vi "FPGA.vi"() -> ()   [LabVIEW 2014]
uses:
  <vilib>/eio/EIONode/EIONode.xnode
  <vilib>/rvi/eio/common/nirviEmuTemplateMethod_errors.vi
panel:
  out "AI5":fxp<+/-,24,5>
  out "AI4":fxp<+/-,24,5>
  out "AI3":fxp<+/-,24,5>
  out "AI2":fxp<+/-,24,5>
  in  "AO2":fxp<+/-,20,5>
  in  "AO1":fxp<+/-,20,5>
  out "AI1":fxp<+/-,24,5>
  out "AI0":fxp<+/-,24,5>
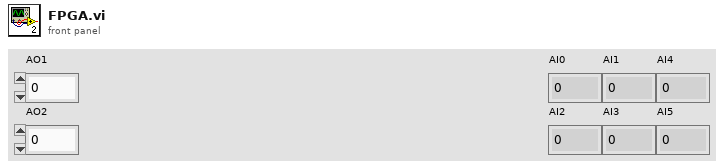
[diagram p1: front panel]
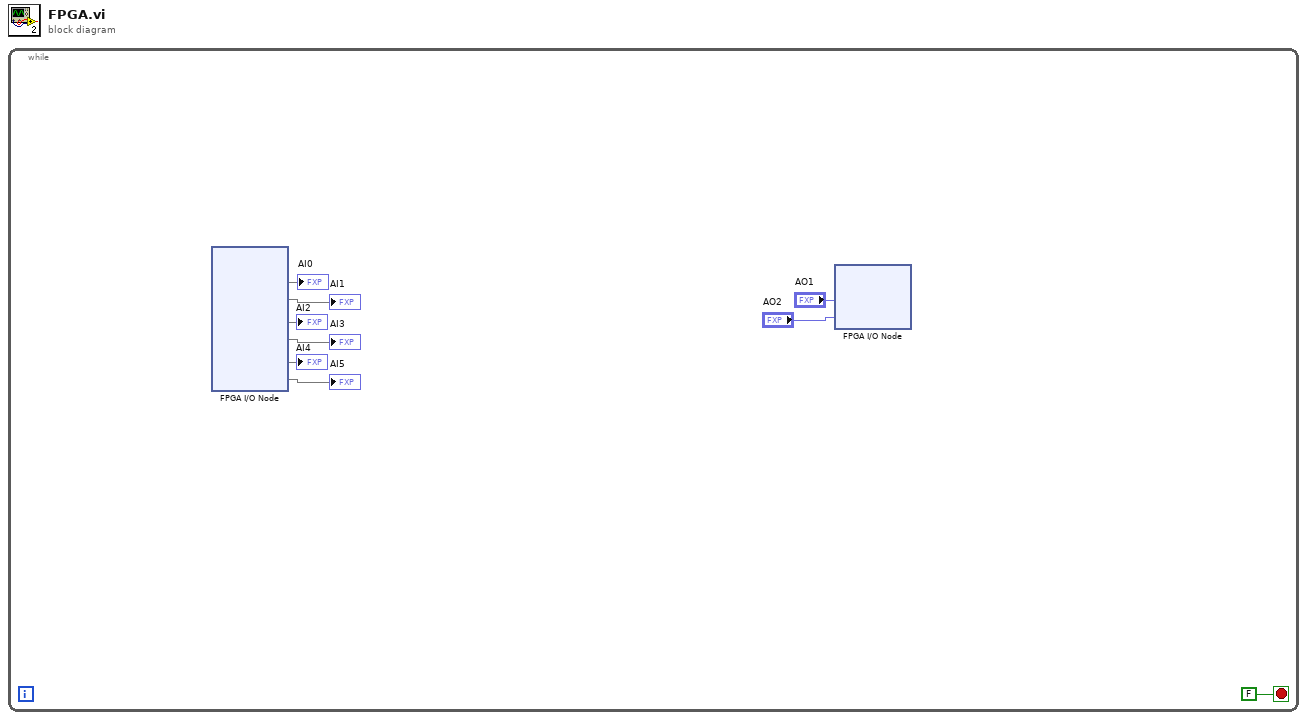
[diagram p0: block diagram]
diagram:
  n1 = while {
    stop <- FALSE stop-if-true
    n2 = xnode "FPGA I/O Node"() -> ("AI0"=→"AI0", "AI1"=→"AI1", "AI2"=→"AI2", "AI3"=→"AI3", "AI4"=→"AI4", "AI5"=→"AI5")  [unwired: 6 in, 6 out]
    n3 = xnode "FPGA I/O Node"("AO1"="AO1", "AO2"="AO2") -> ()  [unwired: 2 in, 2 out]
  }
